vi "Write Cubes.vi"(8 "error in (no error)":errorcluster, 10 "Cubes":refnum<class "Cube.lvclass">[](array[class]), 11 "Cubes in":refnum<class "Cubes.lvclass">) -> (0 "error out":errorcluster, 3 "Cubes out":refnum<class "Cubes.lvclass">)   [LabVIEW 2019, in "22.lvlib" / "Cubes.lvclass"]
uses:
  Cubes.lvclass
  Cube/Cube.lvclass
  Cubes.lvclass/Cubes.ctl
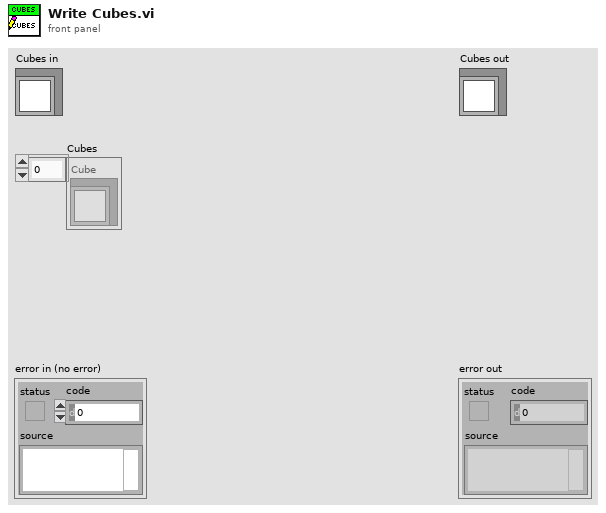
[diagram p1: front panel]
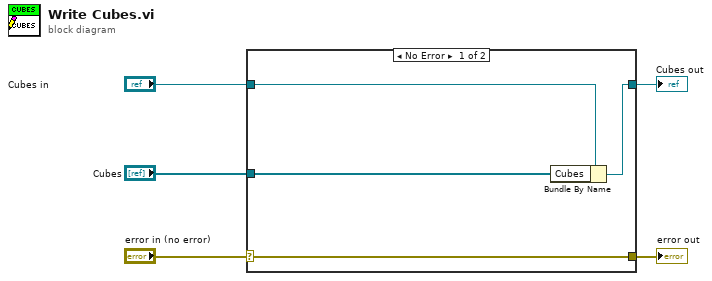
[diagram p0: block diagram]
diagram:
  n1 = case shown="No Error" "error in (no error)" {
    selector: "error in (no error)" -> [w9 w10]
    tunnel: [w9 w10] -> w4
    tunnel: [w7 w11] -> w2
    tunnel: "Cubes in" -> [w8 w11]
    tunnel: "Cubes" -> [w6 _]
    frame No Error {
      n2 = Bundle By Name(cluster=w8, "Cubes"=w6) -> (w7:refnum<class "Cubes.lvclass">)
    }
    frame Error {
    }
  }
  "error out" <- w4
  "Cubes out" <- w2
